vi "树形控件.vi"(0 "长轴M2因子":dbl, 1 "短轴M2因子":dbl, 2 "长轴瑞利长度":dbl, 3 "短轴瑞利长度":dbl, 4 "长轴光束发散角":dbl, 5 "短轴光束发散角":dbl, 6 "长轴束腰位置Z0":dbl, 7 "短轴束腰位置Z0":dbl, 8 "长轴束腰直径":dbl, 10 "短轴束腰直径":dbl, 11 "Tree引用句柄":refnum<vi>) -> ()   [LabVIEW 2015]
panel:
  out "实际项标签（不重复）":string[](array[string])
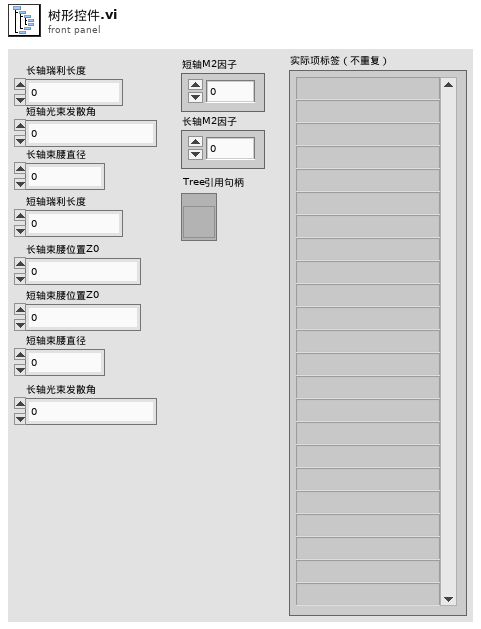
[diagram p1: front panel]
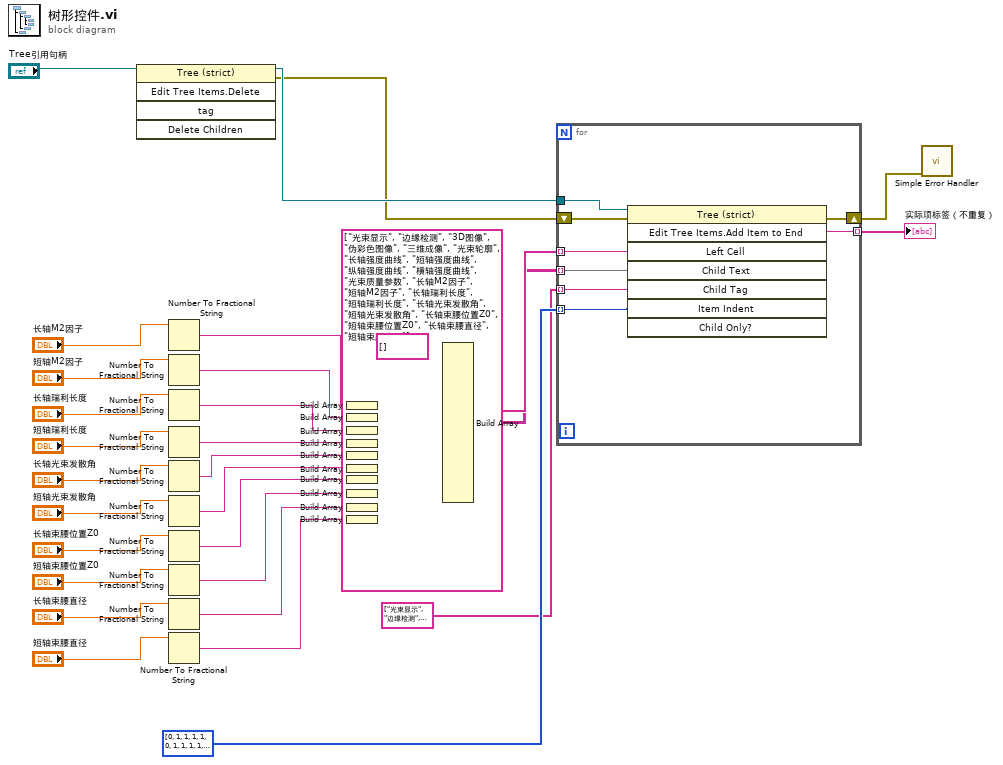
[diagram p0: block diagram]
diagram:
  w5 = string[] [] ("元素")
  n1 = invoke class="Tree (strict)" method="Edit Tree Items.Delete"(reference="Tree引用句柄") -> (reference out=w3:refnum<vi>, error out=w2:errorcluster)  [unwired: 4 in, 3 out]
  n2 = Number To Fractional String(number="长轴M2因子") -> (F-format string=w35:string)  [unwired: 3 in]
  n3 = Number To Fractional String(number="短轴M2因子") -> (F-format string=w34:string)  [unwired: 3 in]
  n4 = Number To Fractional String(number="长轴瑞利长度") -> (F-format string=w33:string)  [unwired: 3 in]
  n5 = Number To Fractional String(number="短轴瑞利长度") -> (F-format string=w32:string)  [unwired: 3 in]
  n6 = Number To Fractional String(number="长轴光束发散角") -> (F-format string=w31:string)  [unwired: 3 in]
  n7 = Number To Fractional String(number="短轴光束发散角") -> (F-format string=w30:string)  [unwired: 3 in]
  n8 = Number To Fractional String(number="长轴束腰位置Z0") -> (F-format string=w29:string)  [unwired: 3 in]
  n9 = Number To Fractional String(number="短轴束腰位置Z0") -> (F-format string=w28:string)  [unwired: 3 in]
  n10 = Number To Fractional String(number="长轴束腰直径") -> (F-format string=w27:string)  [unwired: 3 in]
  n11 = Number To Fractional String(number="短轴束腰直径") -> (F-format string=w26:string)  [unwired: 3 in]
  n12 = Build Array(w35) -> (w25:string[])
  n13 = Build Array(w34) -> (w24:string[])
  n14 = Build Array(w33) -> (w23:string[])
  n15 = Build Array(w32) -> (w22:string[])
  n16 = Build Array(w31) -> (w21:string[])
  n17 = Build Array(w30) -> (w20:string[])
  n18 = Build Array(w29) -> (w19:string[])
  n19 = Build Array(w28) -> (w18:string[])
  n20 = Build Array(w27) -> (w17:string[])
  n21 = Build Array(w26) -> (w16:string[])
  n22 = Build Array(w5, w5, w5, w5, w5, w5, w5, w5, w5, w5, w25, w24, w23, w22, w21, w20, w19, w18, w17, w16) -> (w36:string[][])
  n23 = for {
    tunnel: string[] ["光束显示", "边缘检测", "3D图像", "伪彩色图像", "三维成像", "光束轮廓", "长轴强度曲线", "短轴强度曲线", "纵轴强度曲线", "横轴强度曲线", "光束质量参数", "长轴M2因子", "短轴M2因子", "长轴瑞利长度", "短轴瑞利长度", "长轴光束发散角", "短轴光束发散角", "长轴束腰位置Z0", "短轴束腰位置Z0", "长轴束腰直径", "短轴束腰直径"] ("项名称") -> [w48] mode=indexing
    tunnel: [w41] -> w40 mode=indexing
    tunnel: string[] ["光束显示", "边缘检测", "3D图像", "伪彩色图像", "三维成像", "光束轮廓", "长轴轮廓", "短轴轮廓", "纵轴轮廓", "横轴轮廓", "光束质量参数", "长轴M2因子", "短轴M2因子", "长轴瑞利长度", "短轴瑞利长度", "长轴光束发散角", "短轴光束发散角", "长轴束腰位置Z0", "短轴束腰位置Z0", "长轴束腰直径", "短轴束腰直径"] ("要求的项标签") -> [w46] mode=indexing
    tunnel: i32[] [0, 1, 1, 1, 1, 0, 1, 1, 1, 1, 0, 1, 1, 1, 1, 1, 1, 1, 1, 1, 1] ("项缩进层次") -> [w45] mode=indexing
    tunnel: w36 -> [w47] mode=indexing
    shift-right: [w43] -> w37
    shift-left: w2 -> [w42]
    tunnel: w3 -> [w44]
    # "填充树形控件项"
    n24 = invoke class="Tree (strict)" method="Edit Tree Items.Add Item to End"(reference=w44, error in=w42, "Left Cell"=w48, "Child Text"=w47, "Child Tag"=w46, "Item Indent"=w45) -> (error out=w43:errorcluster, "Edit Tree Items:Add Item to End"=w41:string)  [unwired: 2 in, 6 out]
  }
  "实际项标签（不重复）" <- w40
  n25 = call <vilib>:"Simple Error Handler.vi"("error in (no error)"=w37) -> ()  [unwired: 4 in, 5 out]
